vi "Temperature Limit.vi"() -> ()   [LabVIEW 2015]
doc: "This VI simulates the acquisition of temperature, graphs the temperature, and notifies the user if the temperature is over the limit."
panel:
  in  "Start":bool
  in  "Delta t (ms)":i32(slide)=400 scale=50.0..500.0
  in  "Stop":bool
  in  "High Limit":dbl=28.0 format="%.2f"
  out "Temperature":cluster{"Temperature":dbl, "High Limit":dbl}(graph)={"Temperature"=85.88749999999999, "High Limit"=80.0}
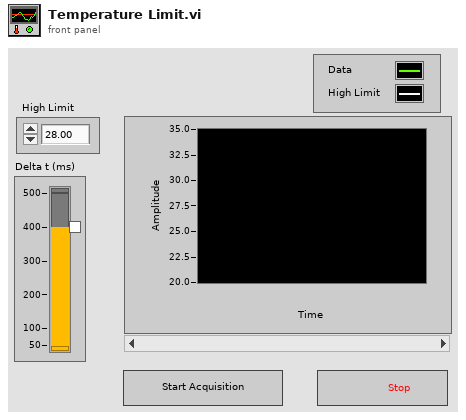
[diagram p1: front panel]
types:
  T1 = enum8{"Enabled", "Disabled", "Disabled and Grayed Out"}
  T2 = cluster{"Temperature Value":dbl, "High Limit":dbl}
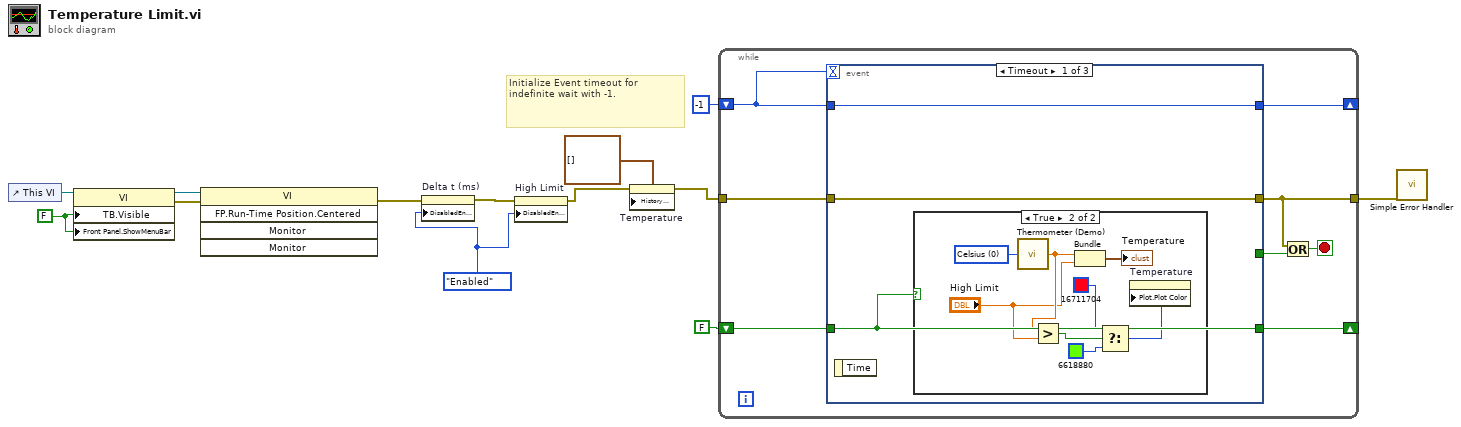
[diagram p0: block diagram]
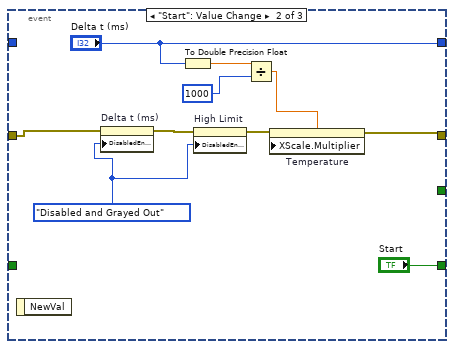
[diagram p3: hidden frame]
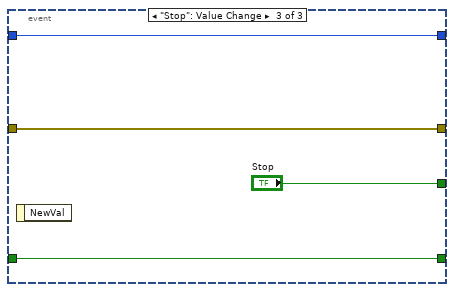
[diagram p4: hidden frame]
diagram:
  w3 = FALSE
  w10 = T1."Enabled" ("Disabled")
  # "Initialize Event timeout for indefinite wait with -1."
  n1 = control-ref of="This VI"() -> (w5:refnum<vi>)
  n2 = property class="VI"(reference=w5, "TB.Visible"=w3, "Front Panel.ShowMenuBar"=w3) -> (reference out=w4:refnum<vi>, error out=w2:errorcluster)  [unwired: 1 in]
  n3 = invoke class="VI" method="FP.Run-Time Position.Centered"(reference=w4, error in=w2) -> (error out=w1:errorcluster)  [unwired: 3 in, 4 out]
  n4 = property on="Delta t (ms)" class="Slide (strict)"(error in=w1, "DisabledEnum"=w10) -> (error out=w9:errorcluster)  [unwired: 1 in, 1 out]
  n5 = property on="High Limit" class="DigNum (strict)"(error in=w9, "DisabledEnum"=w10) -> (error out=w8:errorcluster)  [unwired: 1 in, 1 out]
  n6 = property on="Temperature" class="WFChart (strict)"(error in=w8, "History Data"=cluster{"Temperature":dbl, "High Limit":dbl}[] []) -> (error out=w7:errorcluster)  [unwired: 1 in, 1 out]
  n7 = while {
    tunnel: w7 -> [w21]
    tunnel: [w19] -> w12
    shift-right: [w17] -> _
    shift-left: FALSE ("Start") -> [w16]
    shift-right: [w15] -> _
    shift-left: -1 ("Delta t (ms)") -> [w14]
    stop <- w20 stop-if-true
    n8 = event shown="[0] Timeout" {
      selector: _ -> [_ _ _]
      dyn-events: _ -> [_ _ _]
      timeout: w14 -> [_ _ _]
      tunnel: [_ _ "Stop"] -> w18
      tunnel: w21 -> [w24 w41 w45]
      tunnel: [w24 w38 w45] -> w19
      tunnel: [w22 "Start" w44] -> w17
      tunnel: w16 -> [w22 _ w44]
      tunnel: [w23 "Delta t (ms)" w43] -> w15
      tunnel: w14 -> [w23 _ w43]
      event Timeout {
        n9 = event-data() -> ()  [unwired: 1 in, 1 out]
        n10 = case shown="True" w22 {
          frame False {
          }
          frame True {
            w31 = u16 0 items=["Celsius", "Fahrenheit"] ("Units (0: Celsius)")
            n11 = call "Thermometer (Demo).vi"("Units (0: Celsius)"=w31) -> ("Temperature Value"=w26:dbl)
            n12 = Greater?(x=w26, y="High Limit") -> (0:w27:bool)
            n13 = Bundle("Temperature Value"=w26, "High Limit"="High Limit") -> (→"Temperature":T2)  [unwired: 1 in]
            n14 = Select(t=u32 16711704, s=w27, f=u32 6618880) -> (s? t:f=w28:u32)
            n15 = property on="Temperature" class="WFChart (strict)"("Plot.Plot Color"=w28) -> ()  [unwired: 2 in, 2 out]
          }
        }
      }
      event "Start": Value Change {
        w37 = T1."Disabled and Grayed Out" ("Disabled")
        n16 = event-data() -> ()  [unwired: 1 in, 1 out]
        n17 = property on="Delta t (ms)" class="Slide (strict)"(error in=w41, "DisabledEnum"=w37) -> (error out=w40:errorcluster)  [unwired: 1 in, 1 out]
        n18 = To Double Precision Float(number="Delta t (ms)") -> (double precision float=w35:dbl)
        n19 = property on="High Limit" class="DigNum (strict)"(error in=w40, "DisabledEnum"=w37) -> (error out=w39:errorcluster)  [unwired: 1 in, 1 out]
        n20 = Divide(x=w35, y=1000) -> (x/y=w33:dbl)
        n21 = property on="Temperature" class="WFChart (strict)"(error in=w39, "XScale.Multiplier"=w33) -> (error out=w38:errorcluster)  [unwired: 1 in, 1 out]
      }
      event "Stop": Value Change {
        n22 = event-data() -> ()  [unwired: 1 in, 1 out]
      }
    }
    n23 = Or(x=w19, y=w18) -> (x .or. y?=w20:bool)
  }
  n24 = call <vilib>:"Simple Error Handler.vi"("error in (no error)"=w12) -> ()  [unwired: 4 in, 5 out]
